vi "Host.vi"() -> ()   [LabVIEW 2015]
doc: "This application launches and executes the Tag Bus Data framework configuration for the specified target alias. This is a simple example of the framework API functions, but may also be a suitable starting point for a Host UI or Thick Client that is running a local version of the framework."
uses:
  <vilib>/NI/Module Execution Interface/Engine Runtime/Execution States.ctl
  <vilib>/NI/Module Execution Interface/Engine Runtime/Fault.ctl
  <vilib>/NI/Tag Bus Module Framework/runtime/error classification.ctl
  <vilib>/NI/Module Execution Interface/Engine Runtime/Engine Runtime Interface.lvclass
  <vilib>/NI/DCAF/Tag Editor Core/Framework Configuration Classes/target runtime/PL_Target Runtime.lvclass
  <vilib>/NI/Tag Bus Module Framework/runtime/TBM module execution interface.lvclass
panel:
  in  "Target Selection":enum32{"PC1", "PC2"}(radio)
  in  "configuration file path":path
  out "engine status":T4(array[cluster])
  in  "stop":bool
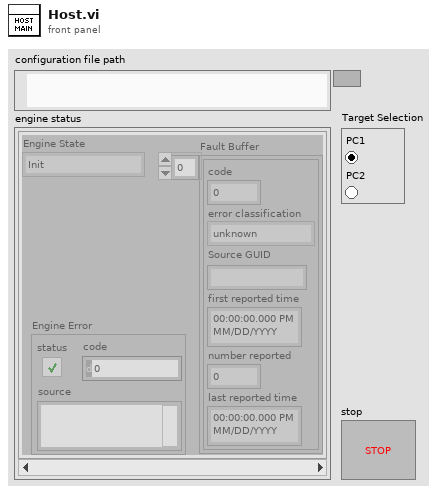
[diagram p1: front panel]
types:
  T1 = typedef "Engine Runtime Interface.lvclass/Execution States.ctl" = enum16{"Init", "Pre-Operational", "Safe-Operational", "Operational", "Stopped"}
  T2 = typedef "Engine Runtime Interface.lvclass/Fault.ctl" = cluster{"code":i32, "error classification":T3, "Source GUID":string, "first reported time":timestamp, "number reported":u32, "last reported time":timestamp}
  T3 = typedef "TBM module execution interface.lvclass/error classification.ctl" = enum16{"unknown", "none", "trivial", "recoverable", "critical"}
  T4 = cluster{"Engine State":T1, "Fault Buffer":T2[], "Engine Error":errorcluster}[]
  T5 = cluster{"Engine State":T1, "Fault Buffer":T2[], "Engine Error":errorcluster}
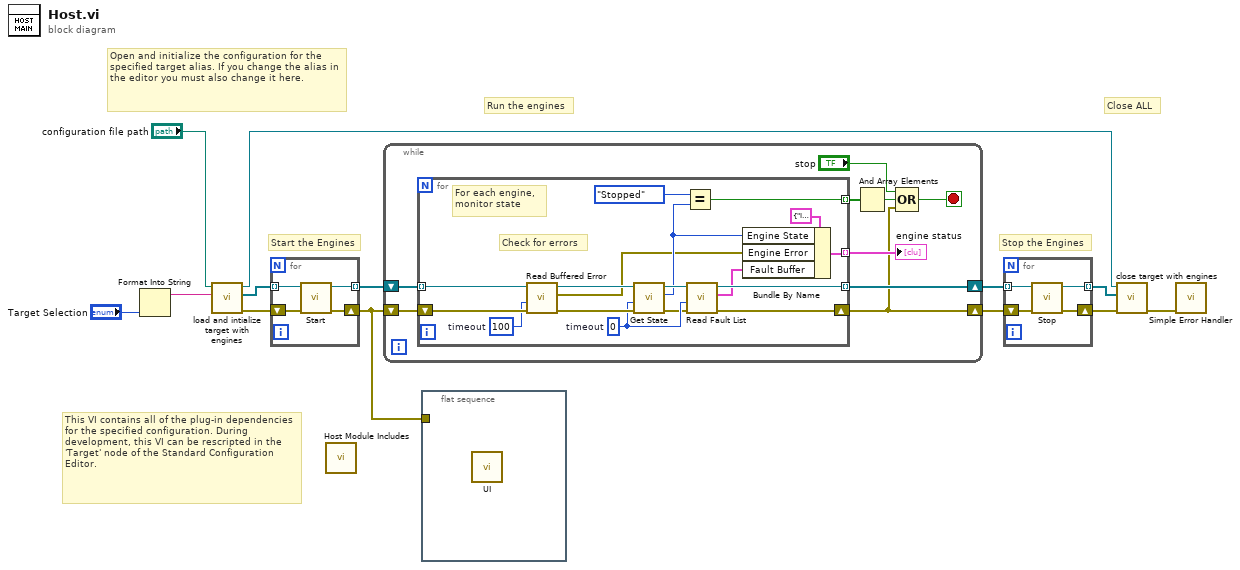
[diagram p0: block diagram]
diagram:
  # "Start the Engines"
  # "Open and initialize the configuration for the specified target alias. If you change the alias in the editor you must also change it here."
  # "Close ALL"
  # "Stop the Engines"
  # "This VI contains all of the plug-in dependencies for the specified configuration. During development, this VI can be rescripted in the 'Target' node of the Standard Configuration Editor."
  # "Run the engines"
  n1 = Format Into String("Target Selection") -> (resulting string=w1:string)  [unwired: 3 in, 1 out]
  n2 = call <vilib>:"load and intialize target with engines.vi"("target alias"=w1, "file path"="configuration file path") -> ("error out"=w10:errorcluster, "engine runtime interfaces"=w9:refnum<class "Engine Runtime Interface.lvclass">[], "target runtime"=w7:refnum<class "PL_Target Runtime.lvclass">)  [unwired: 7 in]
  n3 = for {
    tunnel: [w17] -> w13 mode=indexing
    tunnel: w9 -> [w14] mode=indexing
    shift-right: [w16] -> w4
    shift-left: w10 -> [w15]
    n4 = call-dynamic "Start.vi"("error in"=w15, "Engine Runtime Interface in"=w14) -> ("error out"=w16:errorcluster, "Engine Runtime Interface out"=w17:refnum<class "Engine Runtime Interface.lvclass">)  [unwired: 8 in]
  }
  n5 = call "Host Module Includes.vi"() -> ()  [unwired: 12 in]
  n6 = while {
    shift-right: [w24] -> w12
    shift-left: w13 -> [w26]
    shift-right: [w18] -> w11
    shift-left: w4 -> [w25]
    stop <- w22 stop-if-true
    n7 = for {
      tunnel: w26 -> [w43] mode=indexing
      tunnel: [w35] -> w24 mode=indexing
      tunnel: [w38] -> w20 mode=indexing
      shift-right: [w34] -> w18
      shift-left: w25 -> [w42]
      tunnel: [w30] -> w21 mode=indexing
      w33 = 0  # timeout
      w37 = 100  # timeout
      # "For each engine, \nmonitor state"
      # "Check for errors"
      n8 = call-dynamic "Read Buffered Error.vi"("error in"=w42, "timeout in ms (0)"=w37, "Engine Runtime Interface in"=w43) -> ("error out"=w40:errorcluster, "Engine Error"=w28:errorcluster, "Engine Runtime Interface out"=w41:refnum<class "Engine Runtime Interface.lvclass">)  [unwired: 6 in]
      n9 = call-dynamic "Get State.vi"("error in"=w40, "timeout (-1)"=w33, "Engine Runtime Interface in"=w41) -> ("error out"=w27:errorcluster, "Engine State"=w32:T1, "Engine Runtime Interface out"=w36:refnum<class "Engine Runtime Interface.lvclass">)  [unwired: 6 in]
      n10 = Equal?(x=Execution_States."Stopped" ("Engine State"), y=w32) -> (x = y?=w38:bool)
      n11 = call-dynamic "Read Fault List.vi"("error in"=w27, "timeout (-1)"=w33, "Engine Runtime Interface in"=w36) -> ("error out"=w34:errorcluster, "faults"=w31:T2[], "Engine Runtime Interface out"=w35:refnum<class "Engine Runtime Interface.lvclass">)  [unwired: 6 in]
      n12 = Bundle By Name(cluster=T5 {"Engine State"=enum."Init", "Fault Buffer"=[], "Engine Error"={"status"=FALSE, "code"=0, "source"=""}}, "Engine State"=w32, "Engine Error"=w28, "Fault Buffer"=w31) -> (w30:T5)
    }
    "engine status" <- w21
    n13 = And Array Elements(Boolean array=w20) -> (logical AND=w19:bool)
    n14 = Compound Arithmetic op=OR("stop", w19, w18) -> (w22:bool)
  }
  n15 = flat-sequence {
    tunnel: w4 -> [_]
    frame #0 {
      n16 = call "UI.vi"() -> ()  [unwired: 12 in]
    }
  }
  n17 = for {
    tunnel: w12 -> [w47] mode=indexing
    shift-right: [w44] -> w6
    shift-left: w11 -> [w46]
    tunnel: [w45] -> w8 mode=indexing
    n18 = call-dynamic "Stop.vi"("error in"=w46, "Engine Runtime Interface in"=w47) -> ("error out"=w44:errorcluster, "Engine Runtime Interface out"=w45:refnum<class "Engine Runtime Interface.lvclass">)  [unwired: 8 in]
  }
  n19 = call <vilib>:"close target with engines.vi"("error in"=w6, "Engine Runtime Interfaces"=w8, "Target Runtime"=w7) -> ("error out"=w3:errorcluster)  [unwired: 8 in]
  n20 = call <vilib>:"Simple Error Handler.vi"("error in (no error)"=w3) -> ()  [unwired: 4 in, 5 out]
